vi "DWDT Get Final Time Value.vi"(7 "open interval? (T)":bool=TRUE caption="开区间？(T)", 8 "error in (no error)":errorcluster caption="错误输入（无错误）", 11 "waveform in":digitalwaveform(waveform)={"t0"=timestamp(0 s since 1904-01-01), "dt"=0.0, "Y"={"transitions"=[], "data"=[]}, "error"={"status"=FALSE, "code"=37421928, "source"=""}} caption="波形输入") -> (0 "error out":errorcluster caption="错误输出", 2 "tf":timestamp, 3 "waveform out":digitalwaveform(waveform)={"t0"=timestamp(0 s since 1904-01-01), "dt"=0.0, "Y"={"transitions"=[], "data"=[]}, "error"={"status"=FALSE, "code"=37421928, "source"=""}} caption="波形输出")   [LabVIEW 2018]
doc: "返回<B>波形输入</B>中的结束时间值。 使用的公式为：xf = x0 + <B>波形输入</B>的持续时间。 通过连线数据至<B>波形输入</B>输入端可确定要使用的多态实例，也可手动选择实例。"
panel:
  # "开"
  # "闭"
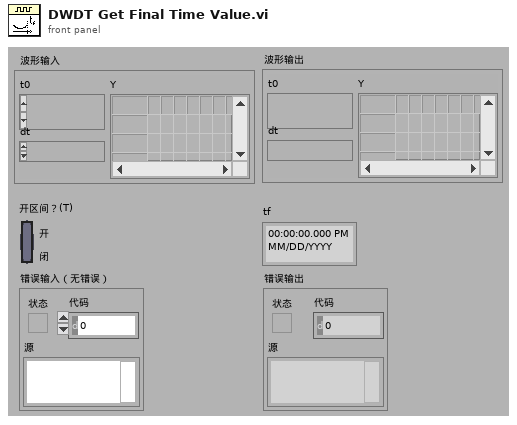
[diagram p1: front panel]
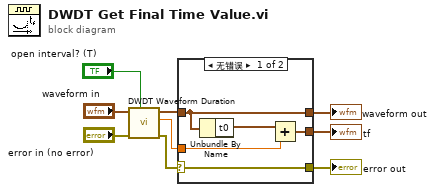
[diagram p0: block diagram]
diagram:
  n1 = call "DWDT Waveform Duration.vi"("open interval? (T)"="open interval? (T)", "error in (no error)"="error in (no error)", "waveform in"="waveform in") -> ("error out"=w2:errorcluster, "duration"=w3:dbl, "waveform out"=w4:digitalwaveform)  [unwired: 6 in]
  n2 = case shown="无错误" w2 {
    selector: w2 -> [w12 w16]
    tunnel: w4 -> [w11 w15]
    tunnel: [w11 w15] -> w8
    tunnel: w3 -> [w14 _]
    tunnel: [w13 _] -> w9
    tunnel: [w12 w16] -> w7
    frame No Error {
      n3 = Unbundle By Name(w11) -> ("t0"=w10:timestamp)
      n4 = Add(x=w10, y=w14) -> (x+y=w13:timestamp)
    }
    frame Error {
    }
  }
  "tf" <- w9
  "waveform out" <- w8
  "error out" <- w7
